vi "Load data from DB.vi"(8 "error in (no error)":errorcluster, 10 "SQL query":string, 11 "Refnum in":T1) -> (0 "error out":errorcluster, 3 "Array":string[][](array[string]))   [LabVIEW 2024, in "DB.lvlib"]
uses:
  DB.lvlib
  <vilib>/addons/database/NI_Database_API.lvlib
  <vilib>/addons/database/Connection.llb/Conn Execute.vi
  <vilib>/addons/database/Recordset.llb/Rec Fetch Recordset Data (R).vi
  <vilib>/addons/database/Connection.llb/Conn ObjectReference.ctl
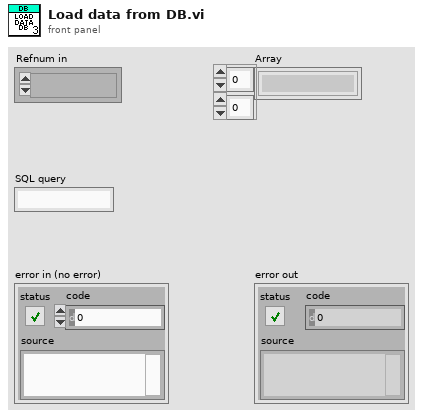
[diagram p1: front panel]
types:
  T1 = typedef "NI_Database_API.lvlib/Conn ObjectReference.ctl" = refnum<k1>
  T2 = typedef "NI_Database_API.lvlib/Rec ObjectReference.ctl" = refnum<k1>
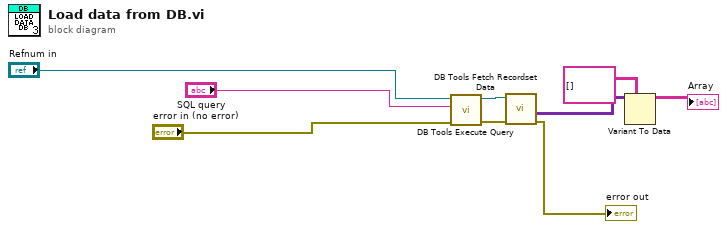
[diagram p0: block diagram]
diagram:
  n1 = call-poly <vilib>:"DB Tools Execute Query.vi"("error in (no error)"="error in (no error)", "SQL query"="SQL query", "connection reference"="Refnum in") -> ("error out"=w8:errorcluster, "recordset reference"=w4:T2)  [unwired: 5 in]
  n2 = call-poly <vilib>:"DB Tools Fetch Recordset Data.vi"("error in (no error)"=w8, "recordset reference"=w4) -> ("error out"=→"error out":errorcluster, "recordset data"=w1:variant[][])  [unwired: 3 in, 1 out]
  n3 = Variant To Data(type=string[][] [], Variant=w1) -> (data=→"Array":string[][])  [unwired: 1 in, 1 out]
